vi "Find Move Locations.vi"(8 "Ocupied array":bool[][](array[boolean]), 11 "Jump Points":set{T1}(c389)) -> (3 "Jump Points":set{T1}(c389))   [LabVIEW 2023]
uses:
  Cluster _Point Location.ctl
panel:
  out "Points to check":T1[](array[typedef])
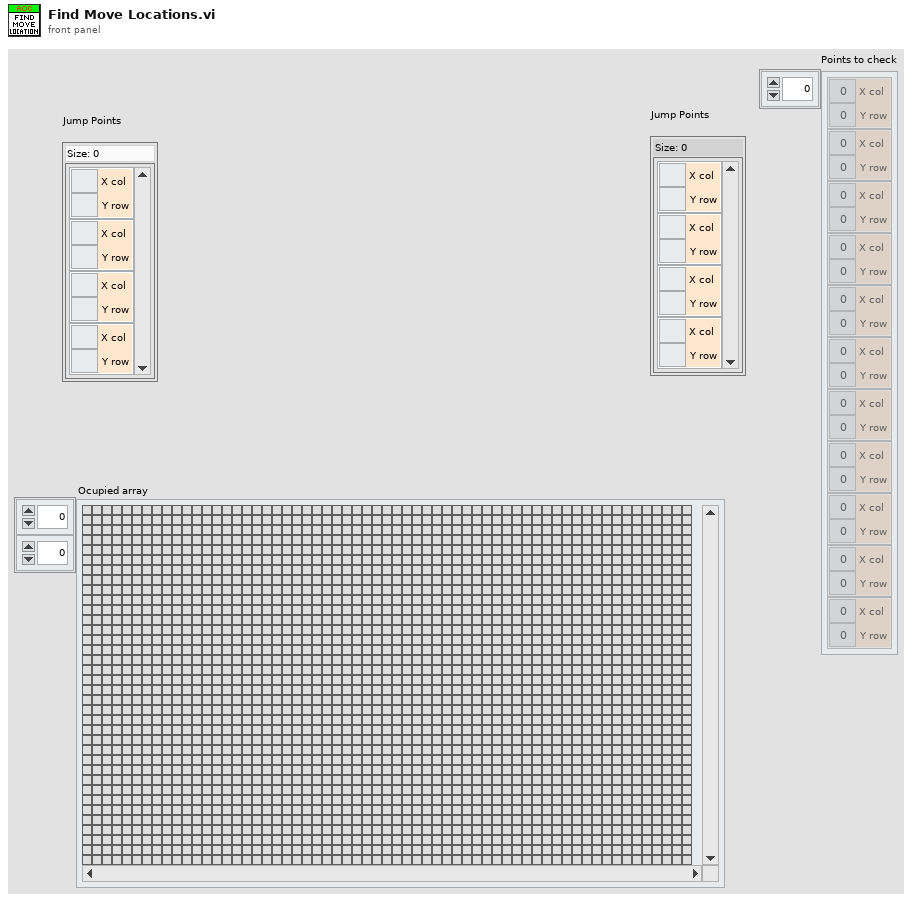
[diagram p1: front panel]
types:
  T1 = typedef "Cluster _Point Location.ctl" = cluster{"X col":i32, "Y row":i32}
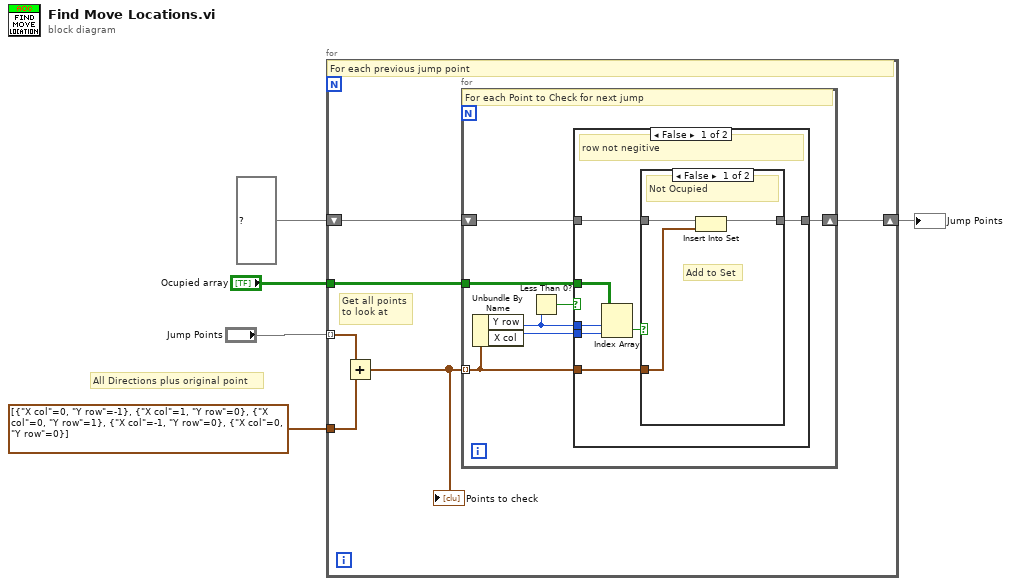
[diagram p0: block diagram]
diagram:
  # "All Directions plus original point"
  n1 = for {
    tunnel: "Jump Points" -> [w11] mode=indexing
    tunnel: T1[] [{"X col"=0, "Y row"=-1}, {"X col"=1, "Y row"=0}, {"X col"=0, "Y row"=1}, {"X col"=-1, "Y row"=0}, {"X col"=0, "Y row"=0}] ("Array") -> [w10]
    shift-right: [w6] -> w1
    shift-left: set{T1} {} ("Jump Points") -> [w7]
    tunnel: "Ocupied array" -> [w8]
    # "Get all points\nto look at"
    # "For each previous jump point"
    n2 = Add(x=w11, y=w10) -> (x+y=w9:T1[])
    "Points to check" <- w9
    n3 = for {
      tunnel: w9 -> [w12] mode=indexing
      tunnel: w8 -> [w18]
      shift-right: [w13] -> w6
      shift-left: w7 -> [w16]
      # "For each Point to Check for next jump"
      n4 = Unbundle By Name(w12) -> ("Y row"=w15:i32, "X col"=w17:i32)
      n5 = Less Than 0?(x=w15) -> (x < 0?=w14:bool)
      n6 = case shown="False" w14 {
        tunnel: w18 -> [w25 _]
        tunnel: w17 -> [w24 _]
        tunnel: w16 -> [w22 w30]
        tunnel: w15 -> [w21 _]
        tunnel: [w19 w30] -> w13
        tunnel: w12 -> [w20 _]
        frame False {
          # "row not negitive"
          n7 = Index Array(array=w25, index (row)=w21, index (col)=w24) -> (element=w23:bool)
          n8 = case shown="False" w23 {
            tunnel: w22 -> [w28 w29]
            tunnel: w20 -> [w26 _]
            tunnel: [w27 w29] -> w19
            frame False {
              # "Add to Set"
              # "Not Ocupied"
              n9 = Insert Into Set(10:w26, 11:w28) -> (3:w27:set{T1})  [unwired: 1 out]
            }
            frame True {
              # "ocupied"
            }
          }
        }
        frame True {
          # "row negitive"
        }
      }
    }
  }
  "Jump Points" <- w1
